vi "is handle valid.vi"(8 "error in (no error)":errorcluster, 11 "MultiUsrp in":refnum<class "MultiUsrp.lvclass">) -> (0 "error out":errorcluster, 3 "MultiUsrp out":refnum<class "MultiUsrp.lvclass">)   [LabVIEW 2023, in "uhd.lvlib" / "MultiUsrp.lvclass"]
uses:
  <userlib>/uhd/MultiUsrp/MultiUsrp.lvclass
  <userlib>/uhd/MultiUsrp/MultiUsrp.lvclass/MultiUsrp.ctl
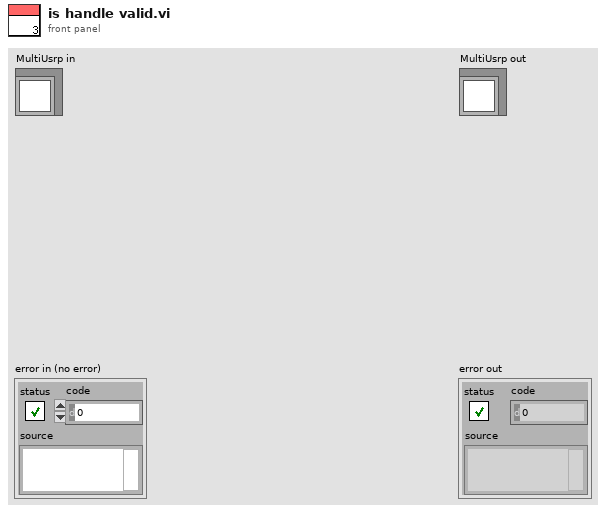
[diagram p1: front panel]
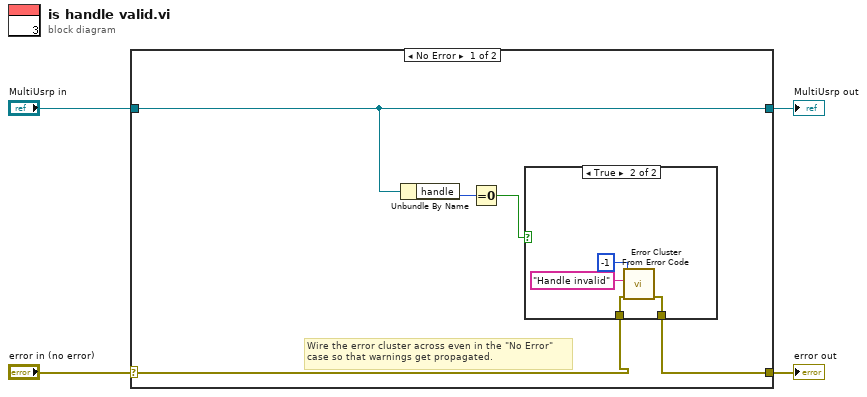
[diagram p0: block diagram]
diagram:
  n1 = case shown="No Error" "error in (no error)" {
    selector: "error in (no error)" -> [w7 w16]
    tunnel: [w6 w16] -> w3
    tunnel: [w9 w15] -> w1
    tunnel: "MultiUsrp in" -> [w9 w15]
    frame No Error {
      # "Wire the error cluster across even in the \"No Error\"\ncase so that warnings get propagated."
      n2 = Unbundle By Name(w9) -> ("handle"=w8:u64)
      n3 = Equal To 0?(x=w8) -> (x = 0?=w5:bool)
      n4 = case shown="True" w5 {
        tunnel: w7 -> [w10 w14]
        tunnel: [w10 w13] -> w6
        frame False {
        }
        frame True {
          n5 = call <vilib>:"Error Cluster From Error Code.vi"("error in (no error)"=w14, "error message (\"\")"="Handle invalid" ("error message (\"\")"), "error code (0)"=-1) -> ("error out"=w13:errorcluster)  [unwired: 6 in]
        }
      }
    }
    frame Error {
    }
  }
  "error out" <- w3
  "MultiUsrp out" <- w1
